vi "Obtain_Variables_and_Deltas.vi"(8 "responsein":string="{\"result\":[[\"intout\",\"stringout\",\"booleanout\",\"doubleout\",\"time\",\"arrayout\"],[0,\"hola\",false,0.000000,17.000000,[0.000000,0.000000]]]}", 11 "expIndex":i32) -> (0 "arraylength":i32, 1 "deltaarray":dbl[][](array[numeric]), 2 "path":string[][](array[string]), 3 "variable array":string[][](array[string]))   [LabVIEW 2020]
uses:
  Configuration/Global_Configurations.vi
panel:
  out "array of clusters":cluster{"path":string[][]}[](array[cluster])
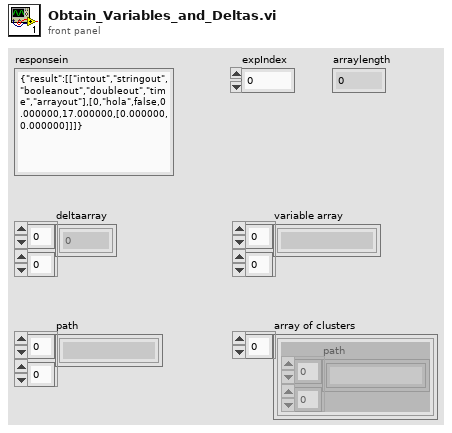
[diagram p1: front panel]
types:
  T1 = cluster{"LabVIEW Host":string, "LabVIEW Port":u16, "Path":path, "Name":string, "Authors":string, "Keywords":string, "Description":string, "Cameras":cluster{"Base URL":string, "Path":string, "Name":string}[], "Sampling":cluster{"Sampled Variable":string, "Delta":dbl}[], "Sampling Freq":u32}[]
  T2 = cluster{"LabVIEW Host":string, "LabVIEW Port":u16, "Path":path, "Name":string, "Authors":string, "Keywords":string, "Description":string, "Cameras":cluster{"Base URL":string, "Path":string, "Name":string}[], "Sampling":cluster{"Sampled Variable":string, "Delta":dbl}[], "Sampling Freq":u32}
  T3 = cluster{"Sampled Variable":string, "Delta":dbl}[]
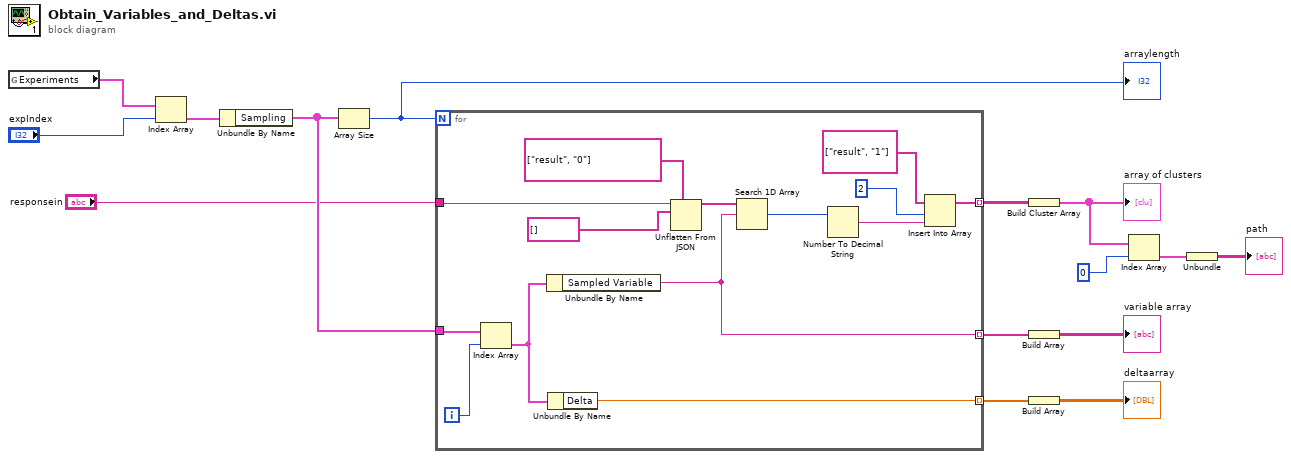
[diagram p0: block diagram]
diagram:
  n1 = global read "Global_Configurations.vi" "Experiments"() -> (w15:T1)
  n2 = Index Array(array=w15, index="expIndex") -> (element=w13:T2)
  n3 = Unbundle By Name(w13) -> ("Sampling"=w12:T3)
  n4 = Array Size(array=w12) -> (size(s)=w4:i32)
  "arraylength" <- w4
  n5 = for {
    N: w4 -> [_]
    tunnel: w12 -> [w29]
    tunnel: "responsein" -> [w23]
    tunnel: [w22] -> w11 mode=indexing
    tunnel: [w21] -> w9 mode=indexing
    tunnel: [w20] -> w3 mode=indexing
    i -> [w17]
    n6 = Index Array(array=w29, index=w17) -> (element=w28:cluster{"Sampled Variable":string, "Delta":dbl})
    n7 = Unbundle By Name(w28) -> ("Sampled Variable"=w20:string)
    n8 = Unbundle By Name(w28) -> ("Delta"=w22:dbl)
    n9 = Unflatten From JSON(path=string[] ["result", "0"], JSON string=w23, type and defaults=string[] [] ("path")) -> (value=w18:string[])  [unwired: 4 in, 1 out]
    n10 = Search 1D Array(1D array=w18, element=w20) -> (index of element=w16:i32)  [unwired: 1 in]
    n11 = Number To Decimal String(number=w16) -> (decimal integer string=w19:string)  [unwired: 1 in]
    n12 = Insert Into Array(array=string[] ["result", "1"] ("path"), index=2, new element=w19) -> (w21:string[])
  }
  n13 = Build Cluster Array(w9) -> (w8:cluster{"path":string[][]}[])
  "array of clusters" <- w8
  n14 = Build Array(w3) -> (→"variable array":string[][])
  n15 = Build Array(w11) -> (→"deltaarray":dbl[][])
  n16 = Index Array(array=w8, index=0) -> (element=w6:cluster{"path":string[][]})
  n17 = Unbundle(w6) -> ("path"=→"path":string[][])
